vi "JJMCclase9.vi"() -> ()   [LabVIEW 2013]
panel:
  out "Potencia":dbl
  out "Exponente":dbl
  out "Base":dbl
  # "generar la base y el exponente con numeros del\n1-10 luego generar la potencia usando el ciclo for"
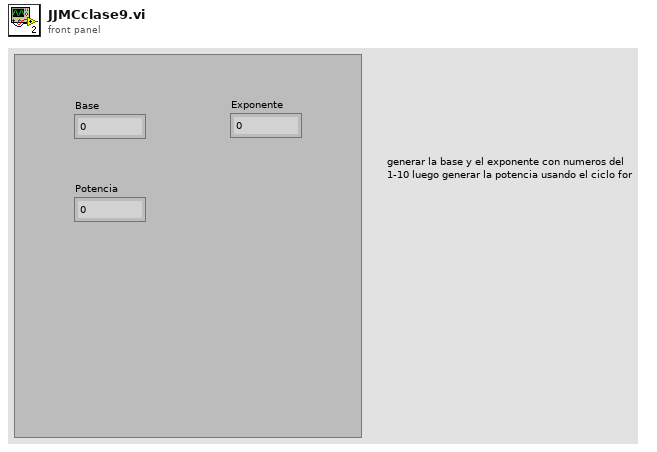
[diagram p1: front panel]
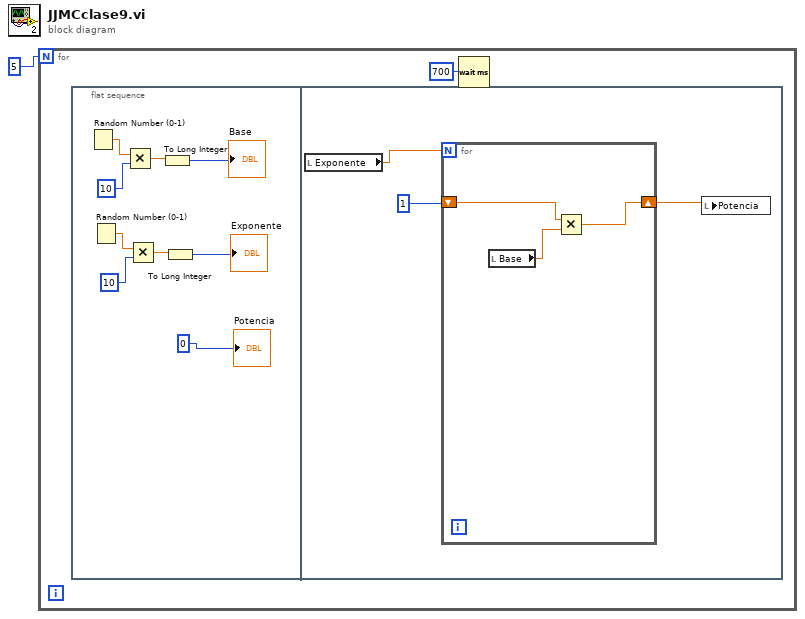
[diagram p0: block diagram]
diagram:
  n1 = for {
    N: 5 -> [_]
    n2 = flat-sequence {
      frame #0 {
        n3 = Random Number (0-1)() -> (number: 0 to 1=w11:dbl)
        n4 = Random Number (0-1)() -> (number: 0 to 1=w5:dbl)
        n5 = Multiply(x=w11, y=10) -> (x*y=w9:dbl)
        n6 = Multiply(x=w5, y=10) -> (x*y=w7:dbl)
        n7 = To Long Integer(number=w9) -> (32bit integer=→"Base":i32)
        n8 = To Long Integer(number=w7) -> (32bit integer=→"Exponente":i32)
        "Potencia" <- 0
      }
      frame #1 {
        n9 = local read "Exponente"() -> (w14:dbl)
        n10 = for {
          N: w14 -> [_]
          shift-right: [w15] -> w12
          shift-left: 1 -> [w16]
          n11 = local read "Base"() -> (w17:dbl)
          n12 = Multiply(x=w16, y=w17) -> (x*y=w15:dbl)
        }
        n13 = local write "Potencia"(w12) -> ()
      }
    }
    n14 = Wait (ms)(milliseconds to wait=700) -> ()  [unwired: 1 out]
  }
